vi "generate filepath.vi"(11 "set file.path GFG (default: T)":bool=TRUE) -> (3 "path":path)   [LabVIEW 2012]
doc: "SciScan 1.2 160622"
uses:
  Custom Controls/file format type def.ctl
  GFG/GFGpathGet.vi
  GFG/GFGstringGet.vi
  GFG/GFG library.lvlib
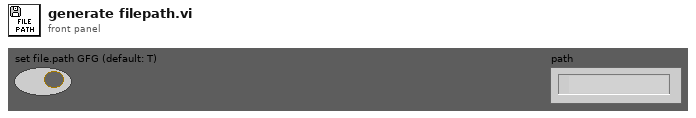
[diagram p1: front panel]
types:
  T1 = typedef "file format type def.ctl" = enum16{"16bit raw", "32bit raw", "16bit multi-tiff (interleave)", "16bit multi-tiff (separate)", "16bit multi-tiff (stacked)", "32bit multi-tiff (interleave)", "32bit multi-tiff (separate)", "32bit multi-tiff (stacked)", "16bit tiff series (interleave)", "16bit tiff series (separate)", "16bit tiff series (stacked)", "32bit tiff series (interleave)", "32bit tiff series (separate)", "32bit tiff series (stacked)"}
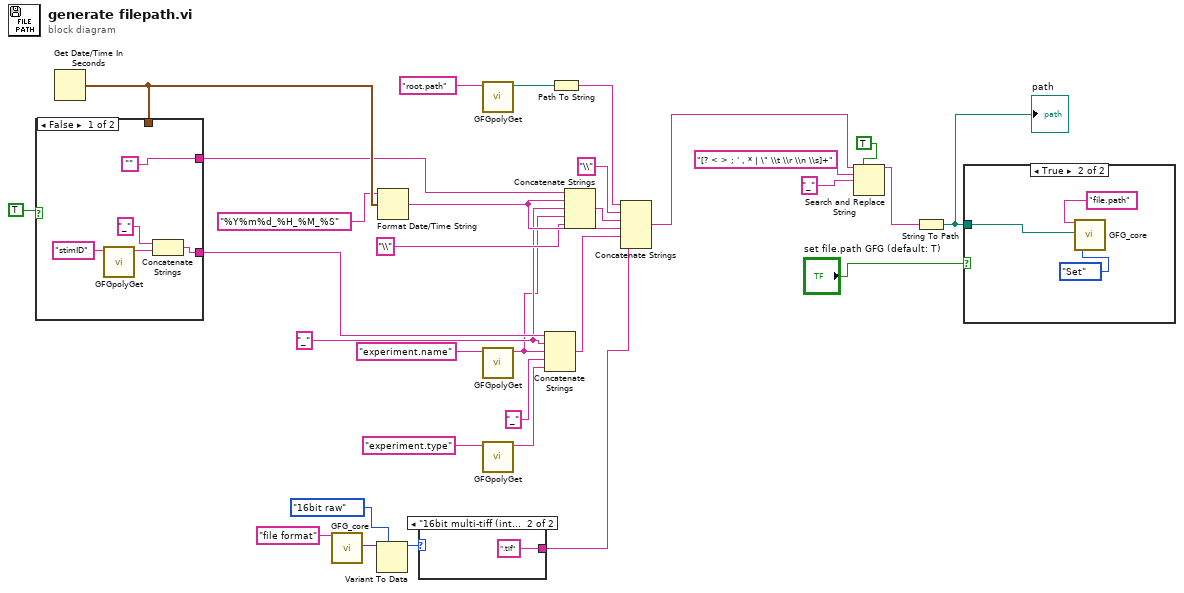
[diagram p0: block diagram]
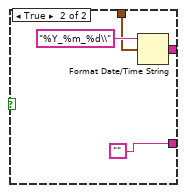
[diagram p3: hidden frame]
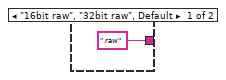
[diagram p4: hidden frame]
diagram:
  w3 = "_" ("string")
  n1 = Get Date/Time In Seconds() -> (seconds since 1Jan1904=w31:timestamp)
  n2 = case shown="False" TRUE {
    tunnel: w31 -> [_ w39]
    tunnel: ["" w38] -> w28
    tunnel: [w32 ""] -> w6
    frame False {
      n3 = call-poly "GFGpolyGet.vi"("Variable Name in"="stimID") -> ("String"=w33:string)  [unwired: 9 in, 1 out]
      n4 = Concatenate Strings("_" ("string"), w33) -> (w32:string)
    }
    frame True {
      n5 = Format Date/Time String(time format string (%c)="%Y_%m_%d\\", seconds (now)=w39) -> (date/time string=w38:string)  [unwired: 1 in]
    }
  }
  n6 = call "GFG_core.vi"("Variable Name in"="file format") -> ("Variant Out"=w21:variant)  [unwired: 12 in, 6 out]
  n7 = Variant To Data(type=file_format_type_def."16bit raw" ("file format"), Variant=w21) -> (data=w15:T1)  [unwired: 1 in, 1 out]
  n8 = Format Date/Time String(time format string (%c)="%Y%m%d_%H_%M_%S", seconds (now)=w31) -> (date/time string=w27:string)  [unwired: 1 in]
  n9 = case shown="\"16bit multi-tiff (interleave)\"..\"32bit tiff series (stacked)\"" w15 {
    tunnel: [".raw" ("string") ".tif" ("string")] -> w14
    frame "16bit raw", "32bit raw", Default {
    }
    frame "16bit multi-tiff (interleave)".."32bit tiff series (stacked)" {
    }
  }
  n10 = call-poly "GFGpolyGet.vi"("Variable Name in"="root.path") -> ("Path"=w25:path)  [unwired: 8 in, 2 out]
  n11 = call-poly "GFGpolyGet.vi"("Variable Name in"="experiment.name") -> ("String"=w2:string)  [unwired: 9 in, 1 out]
  n12 = call-poly "GFGpolyGet.vi"("Variable Name in"="experiment.type") -> ("String"=w17:string)  [unwired: 9 in, 1 out]
  n13 = Concatenate Strings(w6, w3, w2, "_" ("string"), w17) -> (w16:string)
  n14 = Path To String(path=w25) -> (string=w19:string)
  n15 = Concatenate Strings(w28, w27, w3, w2, "\\" ("string")) -> (w30:string)
  n16 = Concatenate Strings(w19, "\\" ("string"), w30, w27, w16, w14) -> (w9:string)
  n17 = Search and Replace String(replace all?=TRUE ("replace all? (F)"), input string=w9, search string="[? < > ; ' , * | \" \\t \\r \\n \\s]+", replace string="_" ("replace string (\"\")")) -> (result string=w8:string)  [unwired: 4 in, 3 out]
  n18 = String To Path(string=w8) -> (path=w13:path)
  "path" <- w13
  n19 = case shown="True" "set file.path GFG (default: T)" {
    tunnel: w13 -> [_ w43]
    frame False {
    }
    frame True {
      n20 = call "GFG_core.vi"("Variable Name in"="file.path" ("Tag in"), "Variant in"=w43, "Action"=enum16{"Init", "Set", "Get"}."Set") -> ()  [unwired: 10 in, 7 out]
    }
  }
